vi "Transform error.vi"(8 "error in (no error)":errorcluster, 9 "server errors":u8[](array[numeric]), 10 "return code":u8, 11 "client in":refnum<class "Generic Client.lvclass">) -> (0 "error out":errorcluster, 1 "server errors out":u8[](array[numeric]), 2 "return code out":u8, 3 "client out":refnum<class "Generic Client.lvclass">)   [LabVIEW 2020, in "NI_SSH.lvlib" / "Generic Client.lvclass"]
uses:
  <vilib>/net/SSH/Client/Generic/Generic Client.lvclass
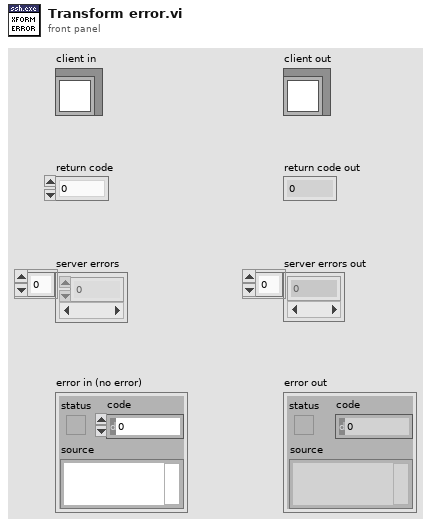
[diagram p1: front panel]
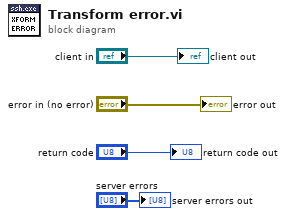
[diagram p0: block diagram]
diagram:
  "error out" <- "error in (no error)"
  "client out" <- "client in"
  "server errors out" <- "server errors"
  "return code out" <- "return code"
